vi "Set3RegsLowLevel_Sylap.vi"(8 "error in (no error)":errorcluster, 9 "Input Value":u64 format="%x", 10 "Reg":u16(ring) items=["TotalOffsetCoarse"=1, "PulseLength"=2, "LaserHalfLength"=3, "LaserMaxCount"=4, "TotalOffset"=17, "ResetCounters"=0, "Reset"=16], 11 "VISA resource name":refnum<visa-resource-name>) -> (0 "error out":errorcluster, 1 "string":string, 2 "appended array":u32[](array[numeric]) format="%x", 3 "VISA resource name out":refnum<visa-resource-name>)   [LabVIEW 2020]
panel:
  out "Reg 2":u16(ring) items=["TotalOffsetCoarse"=1, "PulseLength"=2, "LaserHalfLength"=3, "LaserMaxCount"=4, "TotalOffset"=17, "ResetCounters"=0, "Reset"=16]
  out "return count":u32
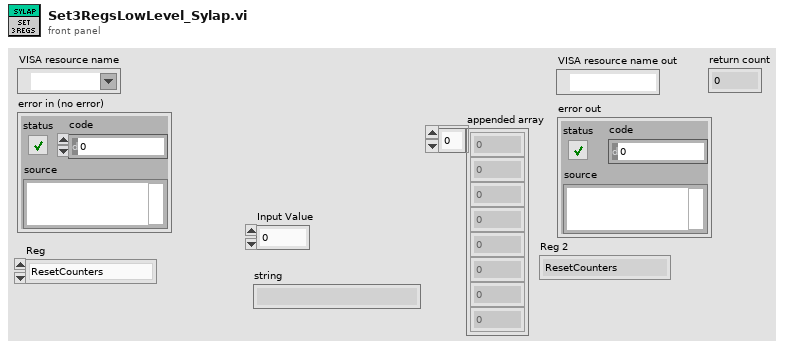
[diagram p1: front panel]
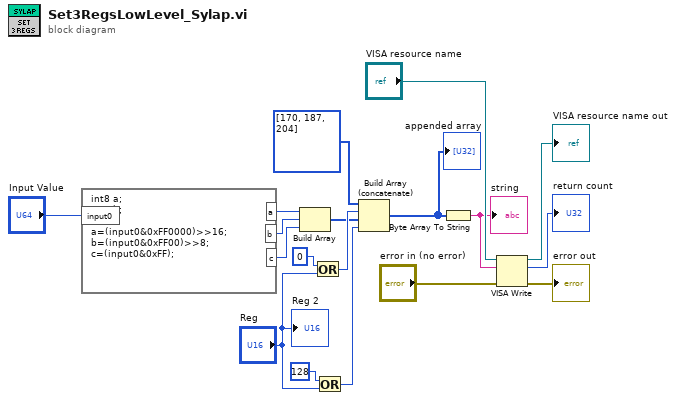
[diagram p0: block diagram]
diagram:
  n1 = formula code="int8 a;\nint8 b;\nint8 c;\na=(input0&0xFF0000)>>16;\nb=(input0&0xFF00)>>8;\nc=(input0&0xFF);"("input0"="Input Value") -> ("a"=w12:i8, "b"=w11:i8, "c"=w10:i8)
  n2 = Build Array(w12, w11, w10) -> (w9:i8[])
  n3 = Or(x=u32 0, y="Reg") -> (x .or. y?=w16:u32)
  n4 = Or(x=u32 128, y="Reg") -> (x .or. y?=w15:u32)
  n5 = Build Array (concatenate)(u32[] [170, 187, 204] ("unsigned byte array"), w16, w9, w15) -> (w1:u32[])
  "appended array" <- w1
  n6 = Byte Array To String(unsigned byte array=w1) -> (string=w7:string)
  "string" <- w7
  n7 = VISA Write(VISA resource name="VISA resource name", write buffer=w7, error in (no error)="error in (no error)") -> (VISA resource name out=→"VISA resource name out":refnum<visa-resource-name>, return count=→"return count":u32, error out=→"error out":errorcluster)
  "Reg 2" <- "Reg"
